vi "2sComplement_array.vi"(1 "binary":i16[](array[numeric]) format="%012b", 2 "Bit Depth":u16=16) -> (0 "decimal":ext[](array[numeric]))   [LabVIEW 2012]
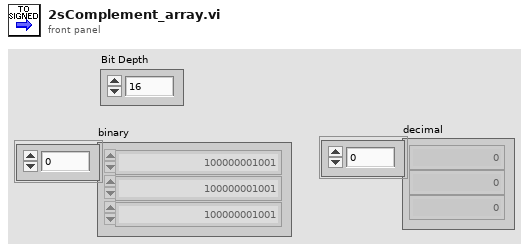
[diagram p1: front panel]
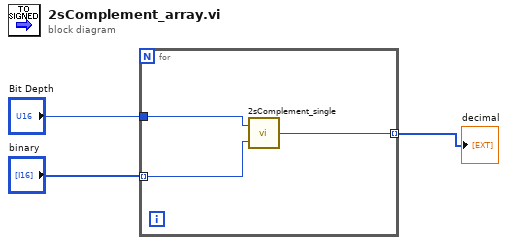
[diagram p0: block diagram]
diagram:
  n1 = for {
    tunnel: "binary" -> [w5] mode=indexing
    tunnel: [w6] -> w2 mode=indexing
    tunnel: "Bit Depth" -> [w4]
    n2 = call "2sComplement_single.vi"("binary"=w5, "Bit Depth"=w4) -> ("Decimal"=w6:i16)
  }
  "decimal" <- w2
